vi "Run Bfr Tx - FIFO Entry Size.vi"(7 "Buffer in":u64, 8 "error in (no error)":errorcluster, 9 "Buffer Size":u64, 11 "Offset in":u64) -> (0 "error out":errorcluster, 1 "Data Size":i32, 3 "Offset out":u64, 4 "Zero Size Detected":bool, 5 "Buffer out":u64, 6 "OOB Detected":bool)   [LabVIEW 2019, in "UDP-Custom-Device Engine.lvlib"]
uses:
  UDP-Custom-Device Engine.lvlib
  <vilib>/NI VeriStand/VeriStand Data/Pointer Operations/Pointer.Read (I32).vi
  <vilib>/NI VeriStand/VeriStand Data/Pointer Operations/Pointer.In-Place Read (I32).vi
  <vilib>/NI VeriStand/VeriStand Data/VeriStand Data.lvlib
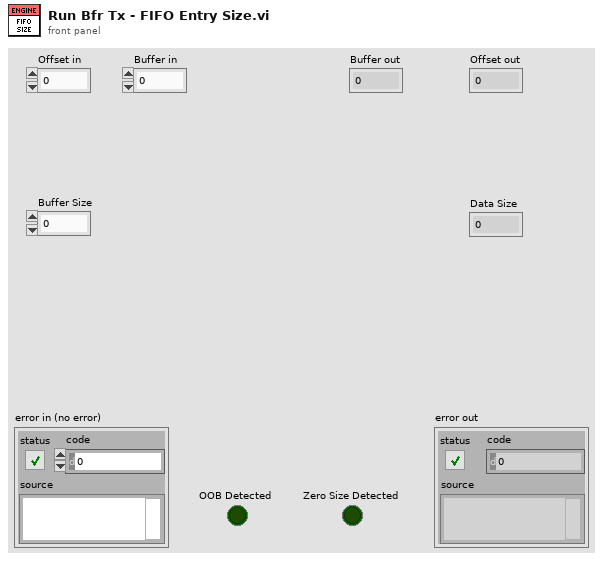
[diagram p1: front panel]
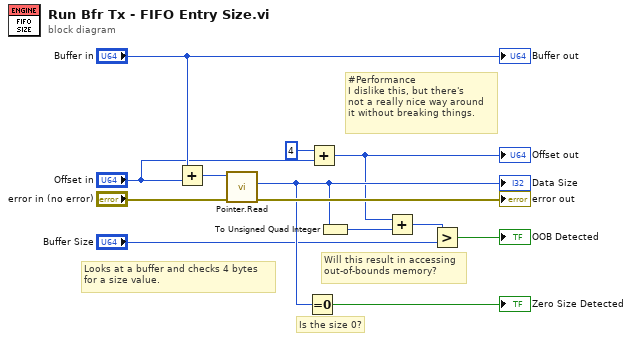
[diagram p0: block diagram]
diagram:
  # "#Performance\nI dislike this, but there's\nnot a really nice way around\nit without breaking things."
  # "Will this result in accessing\nout-of-bounds memory?"
  # "Is the size 0?"
  # "Looks at a buffer and checks 4 bytes\nfor a size value."
  n1 = Add(x="Buffer in", y="Offset in") -> (x+y=w9:u64)
  n2 = call-poly <vilib>:"Pointer.Read.vi"("error in (no error)"="error in (no error)", "pointer in"=w9) -> ("error out"=→"error out":errorcluster, "value"=w6:i32)  [unwired: 7 in, 1 out]
  "Data Size" <- w6
  n3 = Equal To 0?(x=w6) -> (x = 0?=→"Zero Size Detected":bool)
  n4 = Add(x=u64 4, y="Offset in") -> (x+y=w5:u64)
  "Offset out" <- w5
  n5 = To Unsigned Quad Integer(1:w6) -> (0:w4:u64)
  n6 = Add(x=w5, y=w4) -> (x+y=w3:u64)
  n7 = Greater?(x=w3, y="Buffer Size") -> (0:→"OOB Detected":bool)
  "Buffer out" <- "Buffer in"
